vi "SetCommand.vi"(8 "error in (no error)":errorcluster, 11 "PathTokenizer in":refnum<class "PathTokenizer.lvclass">) -> (0 "error out":errorcluster, 3 "PathTokenizer out":refnum<class "PathTokenizer.lvclass">)   [LabVIEW 2019, in "PathTokenizer.lvclass"]
uses:
  PathTokenizer.lvclass
  PathTokenizer.lvclass/PathTokenizer.ctl
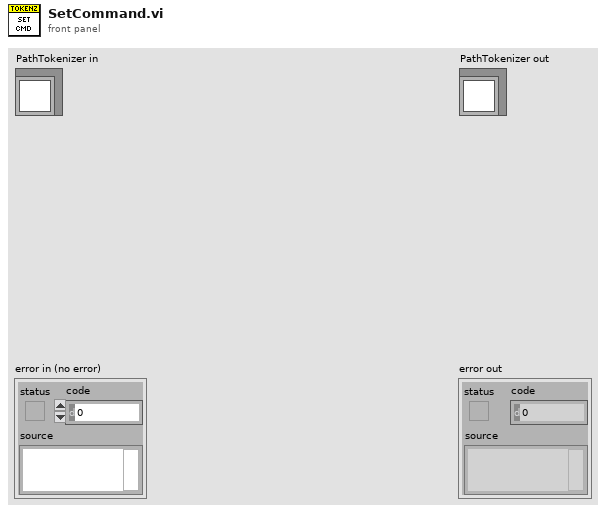
[diagram p1: front panel]
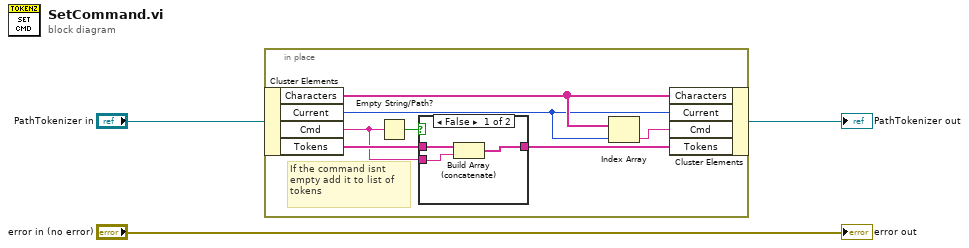
[diagram p0: block diagram]
diagram:
  n1 = in-place {
    # "If the command isnt empty add it to list of tokens"
    n2 = in-place-cluster #1("PathTokenizer in") -> ("Characters"=w10:string[], "Current"=w9:i32, "Cmd"=w4:string, "Tokens"=w5:string[])
    n3 = Empty String/Path?(string/path=w4) -> (empty?=w7:bool)
    n4 = case shown="False" w7 {
      tunnel: [w11 w14] -> w6
      tunnel: w5 -> [w13 w14]
      tunnel: w4 -> [w12 _]
      frame False {
        n5 = Build Array (concatenate)(w13, w12) -> (w11:string[])
      }
      frame True {
      }
    }
    n6 = Index Array(array=w10, index=w9) -> (element=w8:string)
    n7 = in-place-cluster #1("Characters"=w10, "Current"=w9, "Cmd"=w8, "Tokens"=w6) -> (→"PathTokenizer out":refnum<class "PathTokenizer.lvclass">)
  }
  "error out" <- "error in (no error)"
